vi "Cobro.vi"(8 "error in (no error)":errorcluster, 10 "Costo":dbl, 11 "Monedas in":refnum<class "Monedas.lvclass">) -> (0 "error out":errorcluster, 3 "Monedas out":refnum<class "Monedas.lvclass">)   [LabVIEW 2021, in "Monedas.lvlib" / "Monedas.lvclass"]
uses:
  Monedas.lvclass
  Monedas.lvclass/Monedas.ctl
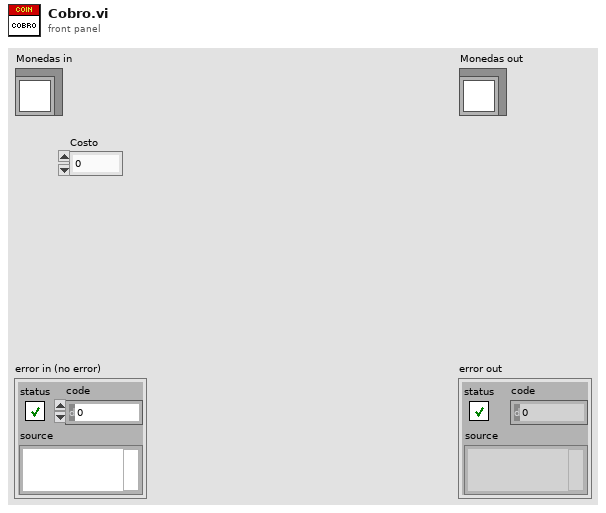
[diagram p1: front panel]
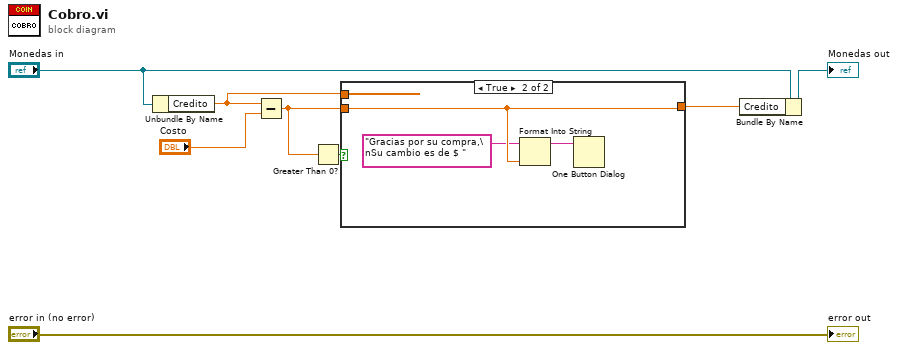
[diagram p0: block diagram]
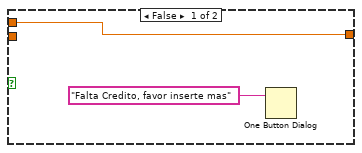
[diagram p2: hidden frame]
diagram:
  n1 = Unbundle By Name("Monedas in") -> ("Credito"=w1:dbl)
  n2 = Subtract(x=w1, y="Costo") -> (x-y=w4:dbl)
  n3 = Greater Than 0?(x=w4) -> (x > 0?=w5:bool)
  n4 = case shown="True" w5 {
    tunnel: w4 -> [_ w13]
    tunnel: [w10 w13] -> w2
    tunnel: w1 -> [w10 _]
    frame False {
      n5 = One Button Dialog(message="Falta Credito, favor inserte mas") -> ()  [unwired: 1 in, 1 out]
    }
    frame True {
      n6 = Format Into String(initial string="Gracias por su compra,\nSu cambio es de $ ", w13) -> (resulting string=w11:string)  [unwired: 2 in, 1 out]
      n7 = One Button Dialog(message=w11) -> ()  [unwired: 1 in, 1 out]
    }
  }
  n8 = Bundle By Name(cluster="Monedas in", "Credito"=w2) -> (→"Monedas out":refnum<class "Monedas.lvclass">)
  "error out" <- "error in (no error)"
